vi "toggle.vi"(1 "Input":bool) -> (0 "Output":bool)   [LabVIEW 2013]
panel:
  in  "Previous State":bool
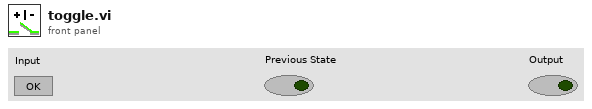
[diagram p1: front panel]
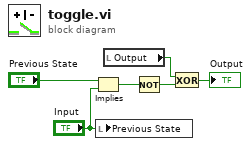
[diagram p0: block diagram]
diagram:
  n1 = Implies(1:"Input", 2:"Previous State") -> (0:w4:bool)
  n2 = local write "Previous State"("Input") -> ()
  n3 = local read "Output"() -> (w3:bool)
  n4 = Not(x=w4) -> (.not. x?=w1:bool)
  n5 = Exclusive Or(1:w1, 2:w3) -> (0:→"Output":bool)
